vi "cast s-64-32 to u64.vi"(11 "fixedpoint_i":fxp<+/-,64,32>) -> (3 "aifxp":u64)   [LabVIEW 2018, in "fixedpoint-cast.lvlib"]
uses:
  <vilib>/rvi/IPIntegrationNode/IPINode_Typedef/niFpgaIPINodeSupportedFamilies.ctl
  <vilib>/rvi/IPIntegrationNode/IPINode_Utilities/niFpgaIPINodeSimCore.vi
  <vilib>/rvi/IPIntegrationNode/IPINode_Xnode/niFpgaIPINode.xnode
  fixedpoint_vhdl/src/cast_s_dash_64_dash_32_to_u64SimFiles/xsim.dir/fixedpoint_to_u64/xsimk6449F698ACB74EA89B6244EDD73F2CE7.dll
  fixedpoint-cast.lvlib
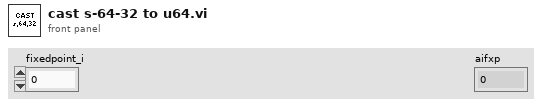
[diagram p1: front panel]
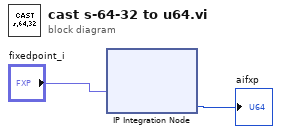
[diagram p0: block diagram]
diagram:
  n1 = xnode "IP Integration Node"("fixedpoint_i"="fixedpoint_i") -> ("u64_o"=→"aifxp":u64)
